vi "teleop drive filter.vi"(10 "input data":T1) -> (2 "output data":T1)   [LabVIEW 2014]
uses:
  TeleopCmd.ctl
  CmdFlag.ctl
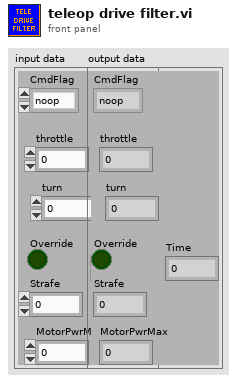
[diagram p1: front panel]
types:
  T1 = typedef "TeleopCmd.ctl" = cluster{"CmdFlag":T2, "throttle":dbl, "turn":dbl, "Override":bool, "Strafe":dbl, "MotorPwrMax":u8, "Time":u32}
  T2 = typedef "CmdFlag.ctl" = enum16{"noop", "logflag", "suspend", "resume"}
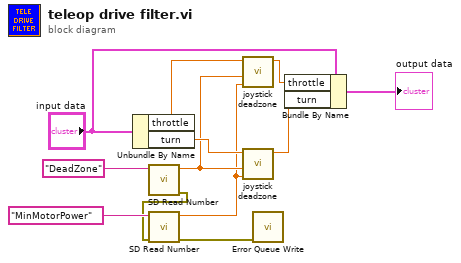
[diagram p0: block diagram]
diagram:
  n1 = Unbundle By Name("input data") -> ("throttle"=w10:dbl, "turn"=w9:dbl)
  n2 = call <vilib>:"SD Read Number.vi"("Name"="DeadZone") -> ("error out"=w2:errorcluster, "Numeric"=w6:dbl)  [unwired: 8 in, 1 out]
  n3 = call <vilib>:"SD Read Number.vi"("error in"=w2, "Name"="MinMotorPower") -> ("error out"=w1:errorcluster, "Numeric"=w5:dbl)  [unwired: 7 in, 1 out]
  n4 = call "joystick deadzone.vi"("minpower"=w5, "deadzone"=w6, "joystick"=w10) -> ("joyout"=w3:dbl)  [unwired: 8 in]
  n5 = call "joystick deadzone.vi"("minpower"=w5, "deadzone"=w6, "joystick"=w9) -> ("joyout"=w4:dbl)  [unwired: 8 in]
  n6 = call "Error Queue Write.vi"("error in (no error)"=w1) -> ()  [unwired: 11 in]
  n7 = Bundle By Name(cluster="input data", "throttle"=w3, "turn"=w4) -> (→"output data":T1)
